vi "triangle wave.vi"(9 "Reset Accumulator_TW":bool, 10 "phase shift":i16, 11 "Frequency":u32=100000) -> (3 "Tri wave out":sgl)   [LabVIEW 2019]
uses:
  <vilib>/rvi/Emulation/niFpgaGetClockAttributes.vi
  <vilib>/rvi/Emulation/niFpgaSctlEmulationGetInTimedLoop.vi
  <vilib>/rvi/Emulation/niFpgaEmulationReportErrorSimple.vi
  <vilib>/rvi/Emulation/niFpgaCriticalErrorInLSC.vi
  <vilib>/rvi/Arithmetic/AddSubMult/XNode/nirviSatArithmetic.xnode
  <vilib>/rvi/FXPMathLib/FxpInterpret/XNode/nifxpmath_Interpret.xnode
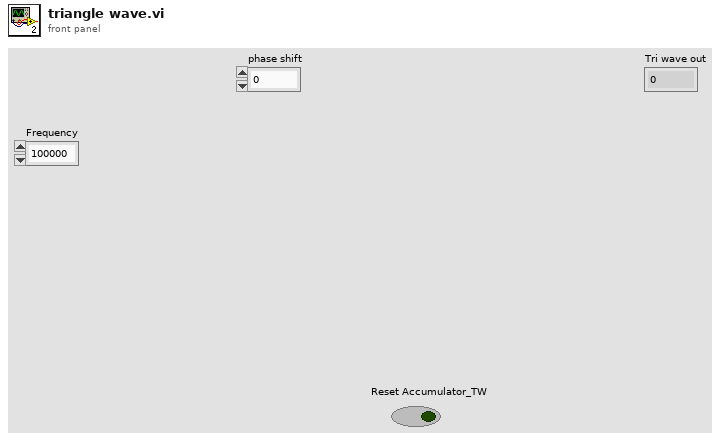
[diagram p1: front panel]
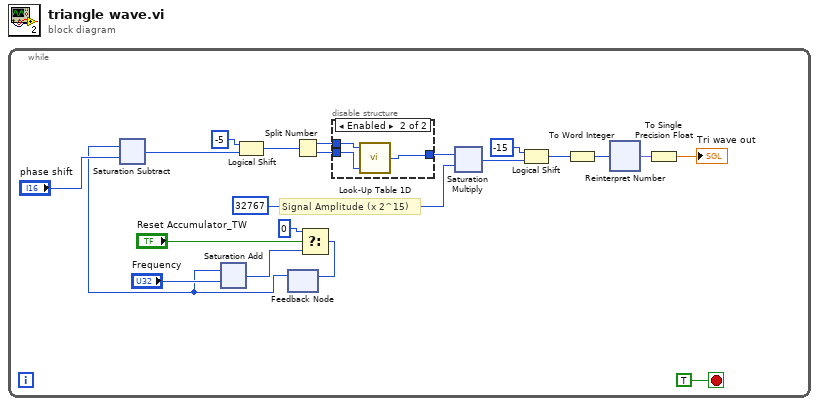
[diagram p0: block diagram]
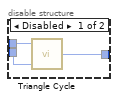
[diagram p2: hidden frame]
diagram:
  n1 = while {
    stop <- TRUE stop-if-true
    # "Signal Amplitude (x 2^15)"
    n2 = feedback #1() -> (w2:u32)  [unwired: 1 in]
    n3 = xnode "Saturation Subtract"("x"=w2, "y"="phase shift") -> ("x-y"=w12:u32)
    n4 = xnode ("Saturation Add")("x"=w2, "y"="Frequency") -> ("x+y"=w16:u32)
    n5 = Logical Shift(y=-5, x=w12) -> (x << y=w18:u32)
    n6 = Split Number(x=w18) -> (hi(x)=w10:u16, lo(x)=w9:u16)
    n7 = Select(t=u32 0, s="Reset Accumulator_TW", f=w16) -> (s? t:f=w17:u32)
    n8 = feedback-in #1(w17) -> ()
    n9 = disable-structure shown="Enabled" {
      disable-tunnel: [w24 w27] -> w11
      disable-tunnel: w10 -> [w23 w26]
      disable-tunnel: w9 -> [w22 w25]
      frame Disabled {
        n10 = call "Triangle Cycle"("address"=w23, "fractional index (x 2^16)"=w22) -> ("data out"=w24:i16)  [unwired: 7 in]
      }
      frame Enabled {
        n11 = call "Look-Up Table 1D"("address"=w26, "fractional index (x 2^16)"=w25) -> ("data out"=w27:i32)  [unwired: 7 in]
      }
    }
    n12 = xnode ("Saturation Multiply")("x"=w11, "y"=i16 32767) -> ("x*y"=w19:i32)
    n13 = Logical Shift(y=-15, x=w19) -> (x << y=w21:i32)
    n14 = To Word Integer(number=w21) -> (16bit integer=w8:i16)
    n15 = xnode "Reinterpret Number"("x"=w8) -> ("y"=w5:fxp<+/-,16,1>)
    n16 = To Single Precision Float(number=w5) -> (single precision float=→"Tri wave out":sgl)
  }
